vi "pin scan.vi"(8 "error in":errorcluster, 10 "data":string, 11 "Users data":T1) -> (0 "error out":errorcluster, 2 "index of element":i32, 3 "User data":T2)   [LabVIEW 2015]
uses:
  Controls/User data.ctl
  Users Data.ctl
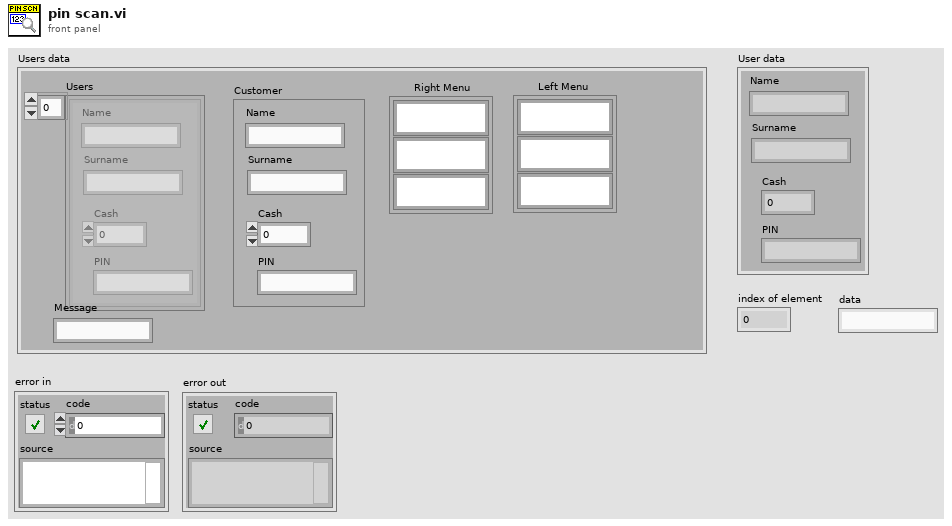
[diagram p1: front panel]
types:
  T1 = typedef "Users Data.ctl" = cluster{"Users":T2[], "Customer":T2, "Message":string, "Right Menu":cluster{"RFS String":string, "RFS String 2":string, "RFS String 3":string}, "Left Menu":cluster{"RFS String":string, "RFS String 2":string, "RFS String 3":string}}
  T2 = typedef "User data.ctl" = cluster{"Name":string, "Surname":string, "Cash":i32, "PIN":string}
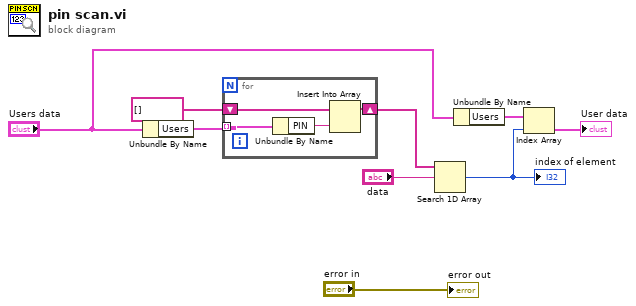
[diagram p0: block diagram]
diagram:
  n1 = Unbundle By Name("Users data") -> ("Users"=w5:T2[])
  n2 = for {
    tunnel: w5 -> [w13] mode=indexing
    shift-right: [w11] -> w3
    shift-left: string[] [] -> [w10]
    n3 = Unbundle By Name(w13) -> ("PIN"=w12:string)
    n4 = Insert Into Array(array=w10, new element=w12) -> (w11:string[])  [unwired: 1 in]
  }
  n5 = Search 1D Array(1D array=w3, element="data") -> (index of element=w8:i32)  [unwired: 1 in]
  "index of element" <- w8
  n6 = Unbundle By Name("Users data") -> ("Users"=w7:T2[])
  n7 = Index Array(array=w7, index=w8) -> (element=→"User data":T2)
  "error out" <- "error in"
